vi "Wyliczanie odległości pomiędzy dwoma punktami.vi"(10 "Polozenie 1":cluster{"X":dbl, "Y":dbl}, 11 "Polozenie in":cluster{"X":dbl, "Y":dbl}) -> (3 "Numeric":dbl)   [LabVIEW 2015, in "Biblioteka moduł map v3.lvlib" / "Matematyczne.lvlib"]
uses:
  Matematyczne.lvlib
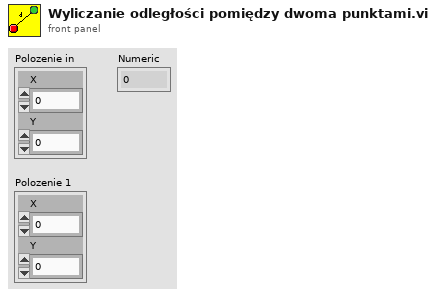
[diagram p1: front panel]
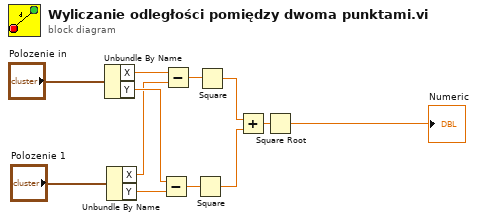
[diagram p0: block diagram]
diagram:
  n1 = Unbundle By Name("Polozenie in") -> ("X"=w3:dbl, "Y"=w5:dbl)
  n2 = Unbundle By Name("Polozenie 1") -> ("X"=w4:dbl, "Y"=w6:dbl)
  n3 = Subtract(x=w5, y=w6) -> (x-y=w7:dbl)
  n4 = Subtract(x=w3, y=w4) -> (x-y=w8:dbl)
  n5 = Square(x=w7) -> (x^2=w10:dbl)
  n6 = Square(x=w8) -> (x^2=w9:dbl)
  n7 = Add(x=w9, y=w10) -> (x+y=w11:dbl)
  n8 = Square Root(x=w11) -> (sqrt(x)=→"Numeric":dbl)
